vi "Build Result File Path.vi"(0 "Charact Result Accessor in":refnum<class "Scalar Charact Result Accessor.lvclass">, 5 "Output Directory":path, 7 "Port 1":string, 9 "Port 2":string, 11 "error in":errorcluster) -> (4 "Charact Result Accessor out":refnum<class "Scalar Charact Result Accessor.lvclass">, 6 "Result File Path":path, 15 "error out":errorcluster)   [LabVIEW 2023, in "RFFixtureCharact.RFPM.lvlib" / "Scalar Charact Result Accessor.lvclass"]
uses:
  Scalar Charact Result Accessor.lvclass
  Base/Charact Result Accessor.lvclass
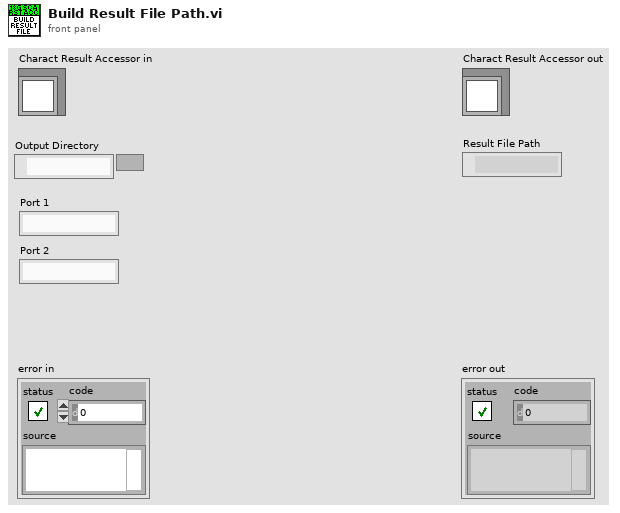
[diagram p1: front panel]
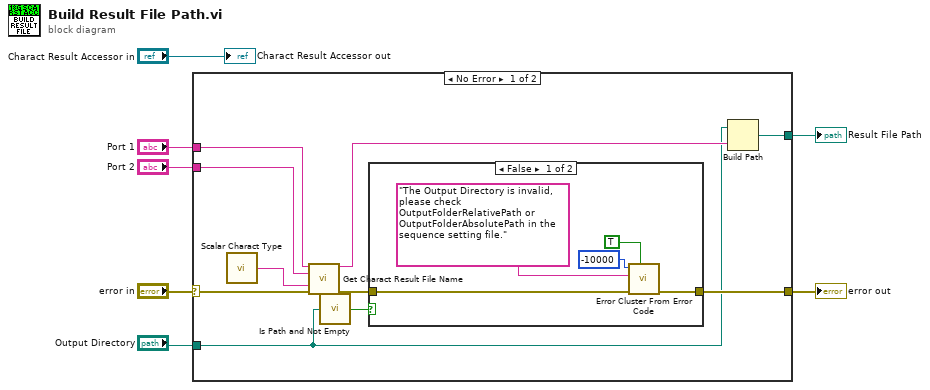
[diagram p0: block diagram]
diagram:
  n1 = case shown="No Error" "error in" {
    selector: "error in" -> [w11 w24]
    tunnel: [w10 w24] -> w6
    tunnel: "Output Directory" -> [w9 _]
    tunnel: "Port 1" -> [w15 _]
    tunnel: "Port 2" -> [w14 _]
    tunnel: [w13 _] -> w2
    frame No Error {
      n2 = call "Scalar Charact Type.vi"() -> ("Charact Type"=w16:string)  [unwired: 1 in]
      n3 = call "Get Charact Result File Name.vi"("Port1"=w15, "Port2"=w14, "Charact Type"=w16, "error in (no error)"=w11) -> ("Charact result file name"=w17:string, "error out"=w8:errorcluster)  [unwired: 10 in]
      n4 = call <vilib>:"Is Path and Not Empty.vi"("path"=w9) -> ("Is Path and Not Empty?"=w12:bool)  [unwired: 4 in]
      n5 = case shown="False" w12 {
        tunnel: w8 -> [w19 w23]
        tunnel: [w18 w23] -> w10
        frame False {
          n6 = call <vilib>:"Error Cluster From Error Code.vi"("show call chain? (False)"=TRUE, "error in (no error)"=w19, "error message (\"\")"="The Output Directory is invalid, please check OutputFolderRelativePath or OutputFolderAbsolutePath in the sequence setting file." ("error message (\"\")"), "error code (0)"=-10000) -> ("error out"=w18:errorcluster)  [unwired: 5 in]
        }
        frame True {
        }
      }
      n7 = Build Path(base path=w9, name or relative path=w17) -> (appended path=w13:path)
    }
    frame Error {
    }
  }
  "error out" <- w6
  "Result File Path" <- w2
  "Charact Result Accessor out" <- "Charact Result Accessor in"
